vi "Icon_Fill in Header.vi"(6 "Box":T1={"Region"={"Left"=0, "Top"=0, "Right"=0, "Bottom"=0, "Width"=0, "Height"=0, "Start"={"Left"=0, "Top"=0}}, "Color"=0, "Fill?"=TRUE}, 8 "Error":errorcluster, 11 "ICON Cluster":T6={"Header"="", "Body"=[], "ImageData"={"image type"=0, "image depth"=0, "image"=[], "mask"=[], "colors"=[], "Rectangle"={"left"=0, "top"=0, "right"=0, "bottom"=0}}, "New Icon"=bytes[0], "Line Status"=[], "Format"={"Color"={"Body txt"=255, "Body Back"=12632256, "Frame"=0, "Header txt"=32768, "Header Back"=16744703, "type"=enum."2 Color"}, "Icon Sizing"={"Rule"=enum."Static", "Header"=TRUE, "Rows"=5, "Width"=32, "Position"=enum."MID-CTR"}}} {"Format"."Icon Sizing"."Rows" min=1 max=5 step=1; "Format"."Icon Sizing"."Width" min=7 max=32 step=1}) -> (0 "Error Out":errorcluster, 3 "ICON Cluster Out":T6={"Header"="", "Body"=[], "ImageData"={"image type"=0, "image depth"=0, "image"=[], "mask"=[], "colors"=[], "Rectangle"={"left"=0, "top"=0, "right"=0, "bottom"=0}}, "New Icon"=bytes[0], "Line Status"=[], "Format"={"Color"={"Body txt"=255, "Body Back"=12632256, "Frame"=0, "Header txt"=32768, "Header Back"=16744703, "type"=enum."2 Color"}, "Icon Sizing"={"Rule"=enum."Static", "Header"=TRUE, "Rows"=5, "Width"=32, "Position"=enum."MID-CTR"}}} {"Format"."Icon Sizing"."Rows" min=1 max=5 step=1; "Format"."Icon Sizing"."Width" min=7 max=32 step=1}, 5 "Output Cluster Out":T4)   [LabVIEW 2014]
doc: "Draws the Header text in the icon"
uses:
  Controls/Cluster/Cluster_Icon Data.ctl
  Controls/String_Picture/STRING_Line Display.ctl
  Controls/Array/String Array_Body Text.ctl
  Controls/Cluster/Cluster_Image Data.ctl
  Controls/Cluster/CLuster_Selectoin Box.ctl
  Controls/String_Picture/Picture_Icon.ctl
  Controls/Cluster/Cluster_Icon Format.ctl
  Controls/Cluster/Cluster_Icon Color Set.ctl
  Controls/Enum/ENUM_Frame Template Select.ctl
  Controls/Cluster/Cluster_Sizing Data.ctl
  Controls/Enum/ENUM_Icon Sizing.ctl
  Controls/Enum/RBENUM_Icon Position.ctl
  Controls/Cluster/CLuster_Line Fit Results.ctl
  Controls/Enum/ENUM RB_Fit Result.ctl
  Controls/Cluster/Cluster_BOX Data.ctl
  Controls/Cluster/Cluster_Region info.ctl
  Controls/Cluster/Cluster_Top Left position.ctl
  Controls/Enum/ENUM_Text Justify.ctl
  Controls/Cluster/Cluster_Text Color Set.ctl
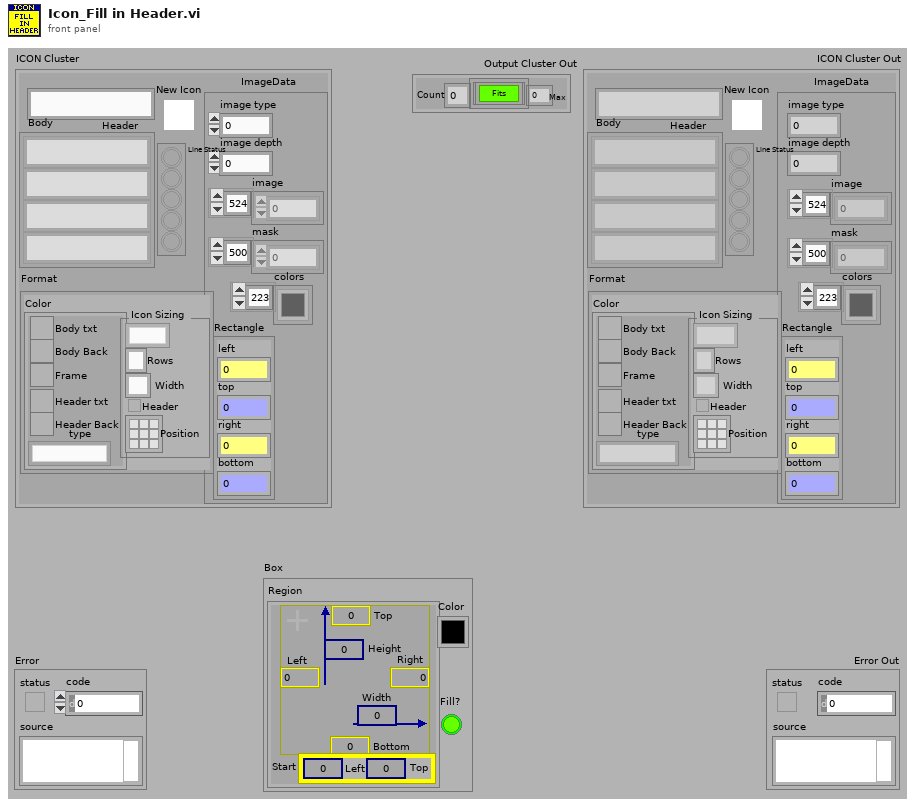
[diagram p1: front panel]
types:
  T1 = typedef "Cluster_BOX Data.ctl" = cluster{"Region":T2, "Color":u32, "Fill?":bool}
  T2 = typedef "Cluster_Region info.ctl" = cluster{"Left":i32, "Top":i32, "Right":i32, "Bottom":i32, "Width":u32, "Height":u32, "Start":T3}
  T3 = typedef "Cluster_Top Left position.ctl" = cluster{"Left":i32, "Top":i32}
  T4 = typedef "CLuster_Line Fit Results.ctl" = cluster{"Fit Result":T5, "Max":i32, "Count":i32}
  T5 = typedef "ENUM RB_Fit Result.ctl" = enum32{"Fits", "Almost Fits", "NO Fit"}
  T6 = typedef "Cluster_Icon Data.ctl" = cluster{"Header":T7, "Body":T8, "ImageData":T9, "New Icon":T11, "Line Status":bool[], "Format":T12}
  T7 = typedef "STRING_Line Display.ctl" = string
  T8 = typedef "String Array_Body Text.ctl" = T7[]
  T9 = typedef "Cluster_Image Data.ctl" = cluster{"image type":i32, "image depth":i32, "image":u8[], "mask":u8[], "colors":u32[], "Rectangle":T10}
  T10 = typedef "CLuster_Selectoin Box.ctl" = cluster{"left":i16, "top":i16, "right":i16, "bottom":i16}
  T11 = typedef "Picture_Icon.ctl" = picture
  T12 = typedef "Cluster_Icon Format.ctl" = cluster{"Color":T13, "Icon Sizing":T15}
  T13 = typedef "Cluster_Icon Color Set.ctl" = cluster{"Body txt":u32, "Body Back":u32, "Frame":u32, "Header txt":u32, "Header Back":u32, "type":T14}
  T14 = typedef "ENUM_Frame Template Select.ctl" = enum16{"2 Color", "5 Color"}
  T15 = typedef "Cluster_Sizing Data.ctl" = cluster{"Rule":T16, "Header":bool, "Rows":u32, "Width":u32, "Position":T17}
  T16 = typedef "ENUM_Icon Sizing.ctl" = enum16{"Static", "Auto"}
  T17 = typedef "RBENUM_Icon Position.ctl" = enum32{"LFT-TOP", "MID-TOP", "RGT-TOP", "LFT-CTR", "MID-CTR", "RGT-CTR", "LFT-BOT", "MID-BOT", "RGT-BOT"}
  T18 = typedef "Cluster_Text Color Set.ctl" = cluster{"BG":u32, "FG":u32}
  T19 = typedef "ENUM_Text Justify.ctl" = enum16{"Left", "Center", "Right"}
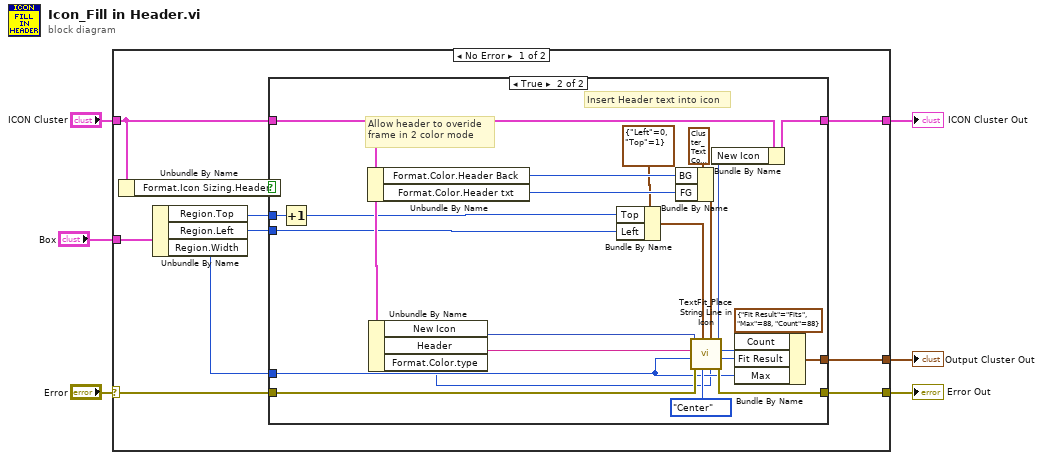
[diagram p0: block diagram]
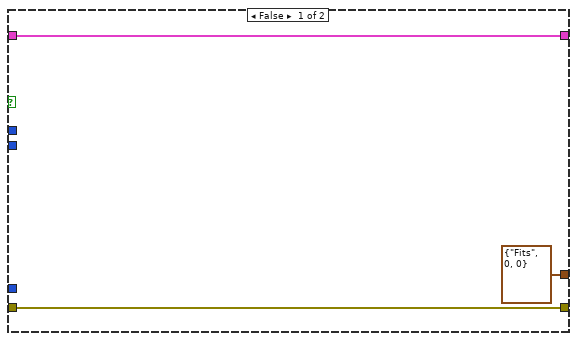
[diagram p2: hidden frame]
diagram:
  n1 = case shown="No Error" "Error" {
    selector: "Error" -> [w13 w43]
    tunnel: [w16 w43] -> w6
    tunnel: "ICON Cluster" -> [w9 w44]
    tunnel: [w15 w44] -> w4
    tunnel: [w14 _] -> w3
    tunnel: "Box" -> [w12 _]
    frame No Error {
      n2 = Unbundle By Name(w9) -> ("Format.Icon Sizing.Header"=w8:bool)
      n3 = Unbundle By Name(w12) -> ("Region.Top"=w7:i32, "Region.Left"=w10:i32, "Region.Width"=w11:u32)
      n4 = case shown="True" w8 {
        tunnel: [w18 w42] -> w16
        tunnel: [w19 w39] -> w15
        tunnel: [T4 {"Fit Result"=enum."Fits", "Max"=0, "Count"=0} ("Cluster") w29] -> w14
        tunnel: w13 -> [w18 w28]
        tunnel: w11 -> [_ w21]
        tunnel: w10 -> [_ w22]
        tunnel: w9 -> [w19 w26]
        tunnel: w7 -> [_ w24]
        frame False {
        }
        frame True {
          # "Allow header to overide\nframe in 2 color mode"
          # "Insert Header text into icon"
          n5 = Increment(x=w24) -> (x+1=w23:i32)
          n6 = Unbundle By Name(w26) -> ("Format.Color.Header Back"=w33:u32, "Format.Color.Header txt"=w34:u32)
          n7 = Unbundle By Name(w26) -> ("New Icon"=w41:T11, "Header"=w37:T7, "Format.Color.type"=w20:T14)
          n8 = Bundle By Name(cluster=T3 {"Left"=0, "Top"=1} ("Starting Positn In"), "Top"=w23, "Left"=w22) -> (w25:T3)
          n9 = Bundle By Name(cluster=T18 {"BG"=128, "FG"=16764108} ("Color Set In"), "BG"=w33, "FG"=w34) -> (w35:T18)
          n10 = call "TextFit_Place String Line in Icon.vi"("Frame"=w20, "Color Set"=w35, "Justify"=ENUM_Text_Justify."Center" ("Justify In"), "Starting Position"=w25, "Error"=w28, "Max Width"=w21, "String"=w37, "ICON"=w41) -> ("Error Out"=w42:errorcluster, "Fit Result Out"=w30:T5, "Final Size Out"=w31:i32, "ICON Out"=w40:T11)
          n11 = Bundle By Name(cluster=w26, "New Icon"=w40) -> (w39:T6)
          n12 = Bundle By Name(cluster=T4 {"Fit Result"=enum."Fits", "Max"=88, "Count"=88} ("Cluster"), "Count"=w31, "Fit Result"=w30, "Max"=w21) -> (w29:T4)
        }
      }
    }
    frame Error {
    }
  }
  "Error Out" <- w6
  "ICON Cluster Out" <- w4
  "Output Cluster Out" <- w3
